vi "Actor Core.vi"(8 "error in":errorcluster, 11 "Thermopower Measurement in":refnum<class "Sequencer Measurement.lvclass">) -> (0 "error out":errorcluster, 3 "Actor out":refnum<class "Actor.lvclass">)   [LabVIEW 2015, in "Sequencer Measurement.lvclass"]
doc: "(<B>Filename</B>: Actor Framework.lvlib:Actor.lvclass:Actor Core.vi)\n\nReceives messages to the actor, reacts to them, and initiates any error handling that may shut the actor down.\n\nDescendant classes may override this VI to append parallel tasks for the actor to complete while it handles messages. Overrides use the Call Parent Method node."
uses:
  Sequencer Measurement.lvclass
  <vilib>/ActorFramework/Actor/Actor.lvclass
  Queued Listbox/Queued Listbox.xctl
  Controls/Menu object.ctl
  Utilities/Increment mode.ctl
  Mag Lab Root/Mag Lab Root.lvclass/Mag Lab Root.ctl
  <vilib>/ActorFramework/Actor/Actor.lvclass/Actor.ctl
  <vilib>/ActorFramework/Message Enqueuer/Message Enqueuer.lvclass/Message Enqueuer.ctl
  Mag Lab Measure Base Messages/Open sub-object parameters Msg/Open nested object parameters Msg.lvclass/Open nested object parameters Msg.ctl
  <vilib>/ActorFramework/Message Enqueuer/Init from Existing Queue.vi
  <vilib>/ActorFramework/Message Enqueuer/Enqueue.vi
  <vilib>/ActorFramework/Message Priority Queue/Priority Enqueue.vi
  Mag Lab Measurement/Mag Lab Measurement.lvclass
  <vilib>/ActorFramework/Message Enqueuer/Message Enqueuer.lvclass
  Mag Lab Measure Base Messages/Open sub-object parameters Msg/Open nested object parameters Msg.lvclass
  Mag Lab Root Messages/Close Front Panel Msg/Close Front Panel Msg.lvclass
  Mag Lab Root/Mag Lab Root.lvclass
panel:
  in  "Settling monitor":T1 {"Object name" items=["Select one"]}
  in  "Parameters":T3={"Mode"=enum."Step", "Start"=0.0, "End"=0.0, "Steps"=2, "Form"=enum."Triangular", "Dwell time"=1.0, "Wait to settle"=FALSE, "Offset compensation"=FALSE, "Offset level"=0.0, "Increment mode"=enum."Linear"}
  in  "Control":T1 {"Object name" items=["Select one"]}
  out "Name":string
  in  "Record":string[](xcontrol)
  in  "Close":bool
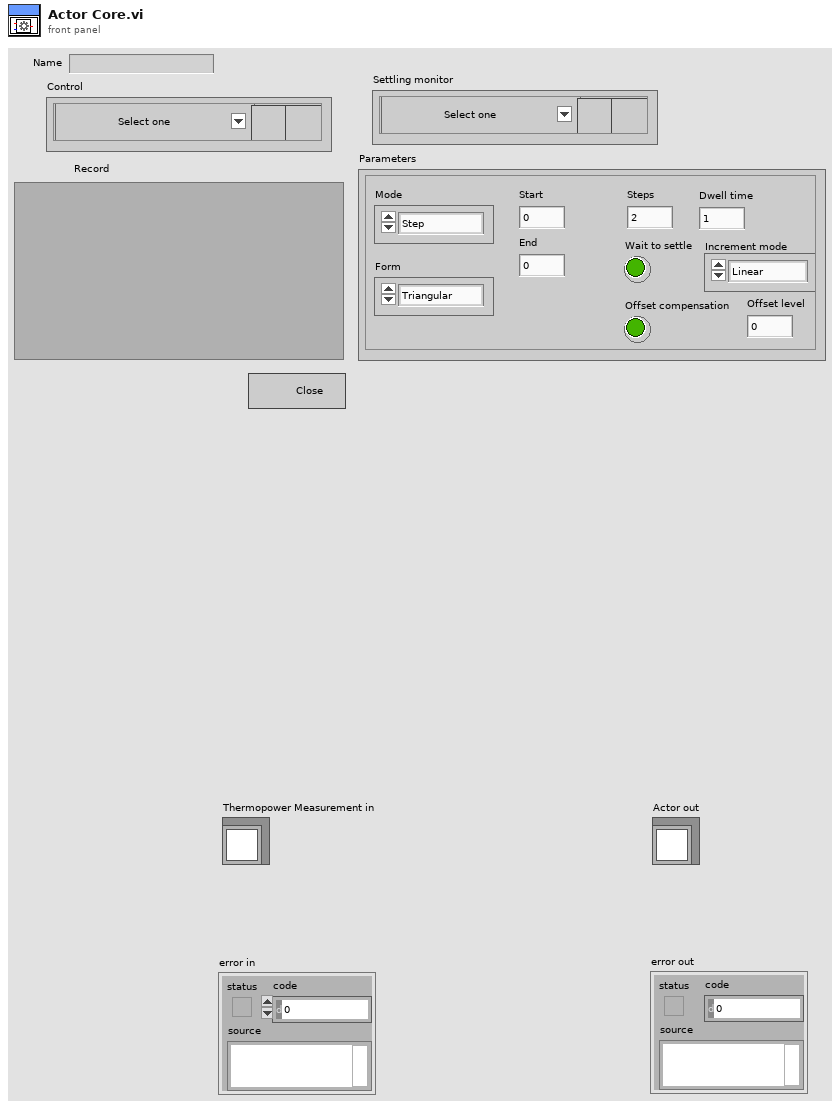
[diagram p1: front panel]
types:
  T1 = typedef "Menu object.ctl" = cluster{"Object name":u16, "Open parameters":bool, "Remove Button":bool}
  T2 = typedef "Increment mode.ctl" = enum16{"Linear", "Square root", "Square", "Log", "Exponent"}
  T3 = cluster{"Mode":enum16{"Sweep", "Step"}, "Start":dbl, "End":dbl, "Steps":i32, "Form":enum16{"Triangular", "Saw tooth"}, "Dwell time":dbl, "Wait to settle":bool, "Offset compensation":bool, "Offset level":dbl, "Increment mode":T2}
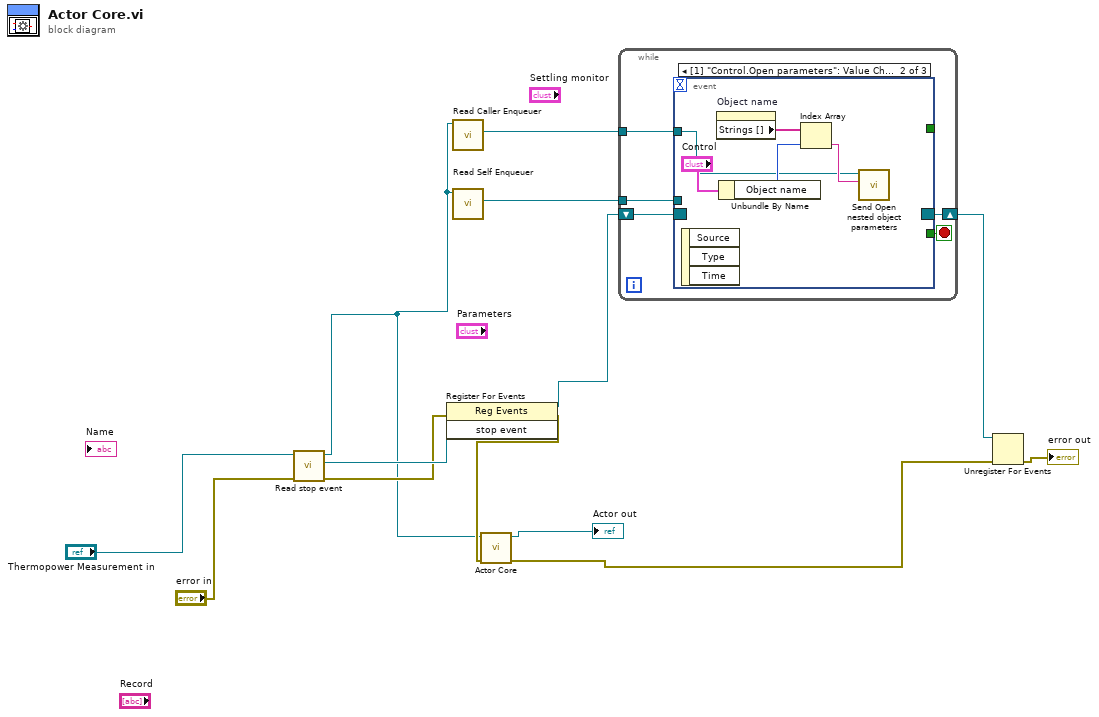
[diagram p0: block diagram]
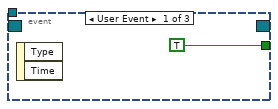
[diagram p2: hidden frame]
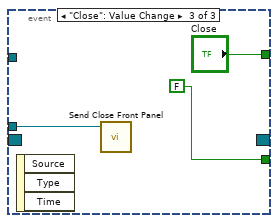
[diagram p3: hidden frame]
diagram:
  n1 = call "Read stop event.vi"("error in (no error)"="error in", "Mag Lab Root in"="Thermopower Measurement in") -> ("error out"=w6:errorcluster, "stop event"=w8:refnum<user-event>, "Mag Lab Root out"=w1:refnum<class "Sequencer Measurement.lvclass">)  [unwired: 7 in]
  n2 = register-events(error in=w6, w8) -> (reference out=w13:refnum<event-registration>, error out=w5:errorcluster)  [unwired: 1 in]
  n3 = call <vilib>:"Read Caller Enqueuer.vi"("Actor"=w1) -> ("Caller Enqueuer"=w11:refnum<class "Message Enqueuer.lvclass">)  [unwired: 10 in]
  n4 = call <vilib>:"Read Self Enqueuer.vi"("Actor"=w1) -> ("Self Enqueuer"=w12:refnum<class "Message Enqueuer.lvclass">)  [unwired: 10 in]
  n5 = call-parent "Actor Core.vi"("error in"=w5, "Mag Lab Measure Base in"=w1) -> ("error out"=w3:errorcluster, "Actor out"=→"Actor out":refnum<class "Actor.lvclass">)  [unwired: 8 in]
  n6 = while {
    tunnel: w12 -> [w16]
    tunnel: w11 -> [w15]
    shift-right: [w14] -> w10
    shift-left: w13 -> [w18]
    stop <- w17 stop-if-true
    n7 = event shown="[1] \"Control.Open parameters\": Value Change" {
      selector: w18 -> [_ _ _]
      dyn-events: [_ _ _] -> w14
      timeout: _ -> [_ _ _]
      tunnel: [TRUE _ FALSE] -> w17
      tunnel: w16 -> [_ _ w26]
      tunnel: w15 -> [_ w20 _]
      tunnel: [_ _ "Close"] -> _
      event User Event {
        n8 = event-data() -> ()  [unwired: 1 in, 2 out]
      }
      event Value Change {
        n9 = event-data() -> ()  [unwired: 1 in, 3 out]
        n10 = property on="Object name" class="Ring (strict)"() -> ("Strings []"=w24:string[])  [unwired: 2 in, 2 out]
        n11 = Unbundle By Name("Control") -> ("Object name"=w23:u16)
        n12 = Index Array(array=w24, index=w23) -> (element=w22:string)
        n13 = call "Send Open nested object parameters.vi"("Object name"=w22, "Message Enqueuer"=w20) -> ()  [unwired: 8 in, 2 out]
      }
      event "Close": Value Change {
        n14 = event-data() -> ()  [unwired: 1 in, 3 out]
        n15 = call "Send Close Front Panel.vi"("Message Enqueuer"=w26) -> ()  [unwired: 9 in, 2 out]
      }
    }
  }
  n16 = Unregister For Events(event registration refnum=w10, error in=w3) -> (error out=→"error out":errorcluster)
